vi "Plantilla.vi"() -> ()   [LabVIEW 2013]
uses:
  <vilib>/Platform/TimedLoop/XDataNode/timing_clust.ctl
  <vilib>/Platform/TimedLoop/XDataNode/nitl_modes.ctl
  <vilib>/Platform/TimedLoop/XDataNode/wakeup.ctl
  <vilib>/platform/TimedLoop/XDataNode/XDataNode.xnode
  <vilib>/Platform/TimedLoop/XDataNode/XDNodeRunTimeDep.lvlib
panel:
  out "Boolean 5":bool
  out "Boolean 4":bool
  in  "Offset Loop B 3":i64=5
  out "Boolean 3":bool
  out "Boolean 2":bool
  out "Boolean":bool
  in  "Offset Loop B 2":i64=5
  out "Timed Loop Iteration Start Times":i64[][](graph)
  in  "Offset Loop B":i64=5
  in  "Offset Loop A":i64
  in  "Period Loop A":i64=10
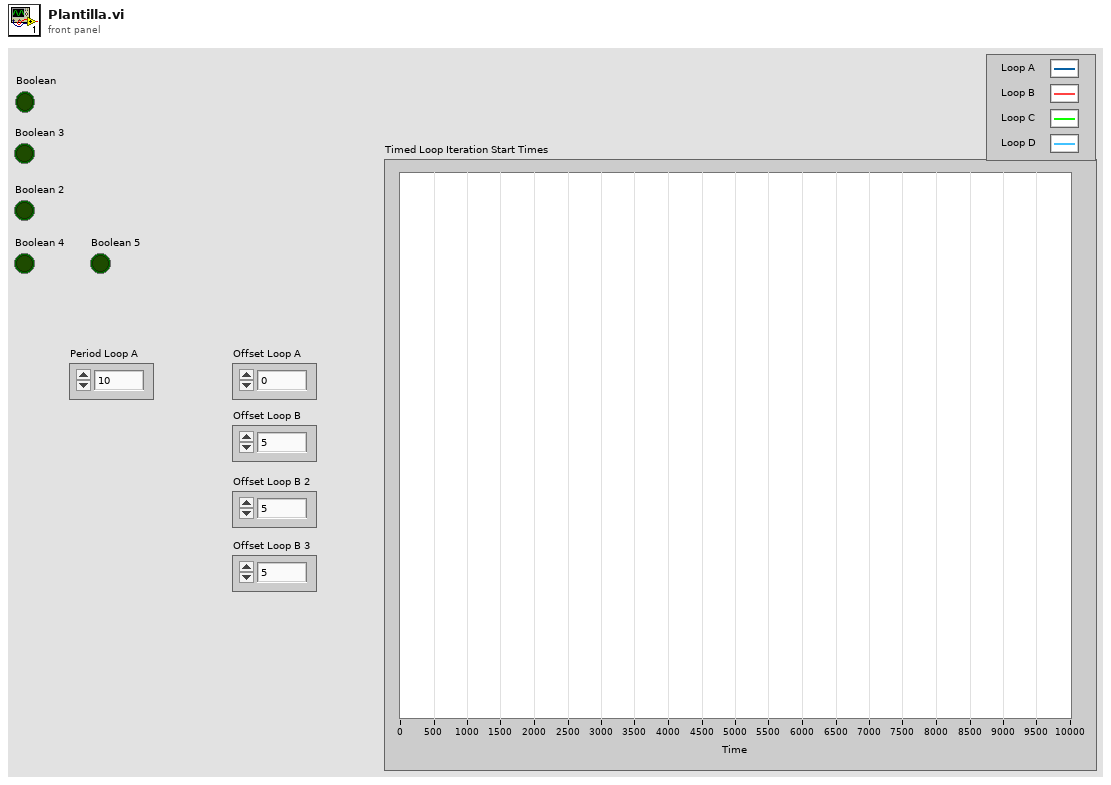
[diagram p1: front panel]
types:
  T1 = typedef "XDNodeRunTimeDep.lvlib/timing_clust.ctl" = cluster{"Expected End [f-1]":u64, "Actual End [f-1]":u64, "Finished Late? [f-1]":bool, "Expected End [i-1]":u64, "Actual End [i-1]":u64, "Finished Late? [i-1]":bool, "Expected Start [i]":u64, "Actual Start [i]":u64, "Expected Start [f]":u64, "Actual Start [f]":u64, "Source Name":string, "Structure Name":string, "Period":i64, "Deadline":i64, "Offset":i64, "Start":i64, "Priority":i32, "Timeout":i32, "Mode":T2, "Wakeup Reason":T3, "Error":errorcluster, "Source Type":string, "Secondary Source Type":string, "Global End Time":u64, "Global Start Time":u64, "Frame Duration":u64, "Iteration Duration":u64, "Assigned CPU":i32, "I/O Scan Engine Mode":u32}
  T2 = typedef "XDNodeRunTimeDep.lvlib/nitl_modes.ctl" = enum32{"No Change", "Process missed periods, maintain original phase", "Discard missed periods, maintain original phase", "Process missed periods, ignore original phase", "Discard missed periods, ignore original phase"}
  T3 = typedef "XDNodeRunTimeDep.lvlib/wakeup.ctl" = enum32{"Normal", "Aborted", "Asynchronous wakeup", "Timing source error", "Timed loop error", "Timeout"}
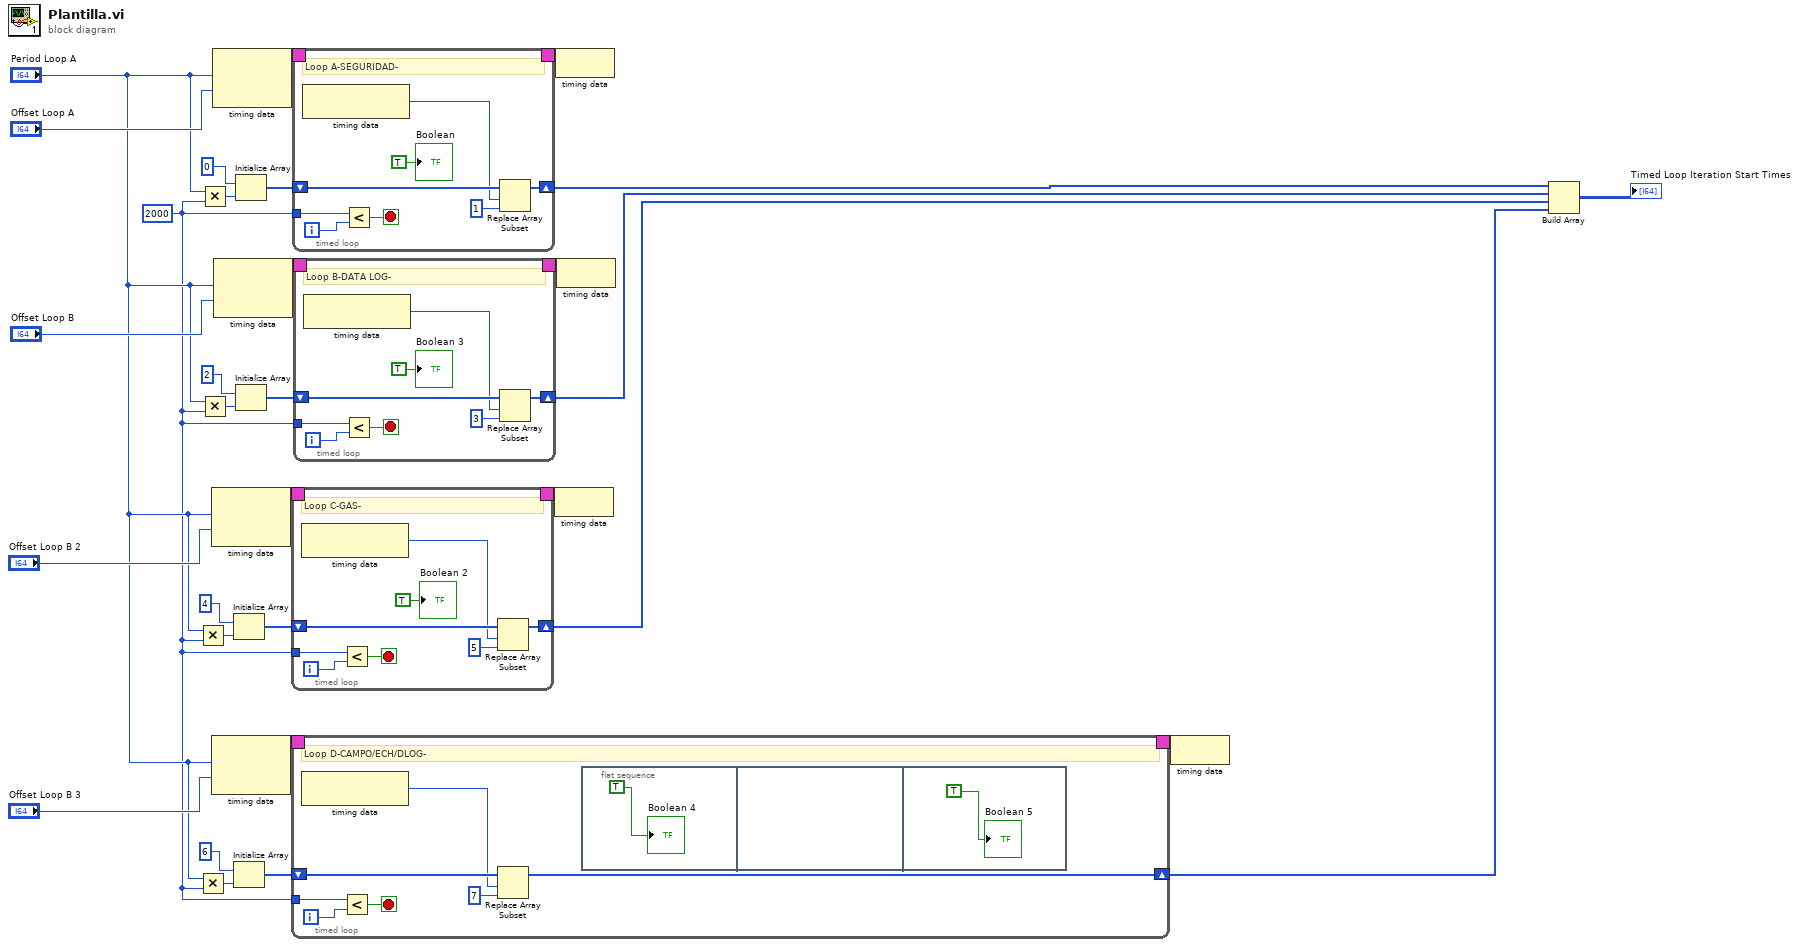
[diagram p0: block diagram]
diagram:
  w1 = i64 2000
  n1 = Multiply(x="Period Loop A", y=w1) -> (x*y=w13:i64)
  n2 = Multiply(x="Period Loop A", y=w1) -> (x*y=w6:i64)
  n3 = Multiply(x="Period Loop A", y=w1) -> (x*y=w25:i64)
  n4 = Multiply(x="Period Loop A", y=w1) -> (x*y=w22:i64)
  n5 = node-c288("Period Loop A", "Offset Loop B 2") -> (w16:T1)
  n6 = node-c288("Period Loop A", "Offset Loop B 3") -> (w9:T1)
  n7 = node-c288("Period Loop A", "Offset Loop A") -> (w29:T1)
  n8 = node-c288("Period Loop A", "Offset Loop B") -> (w31:T1)
  n9 = Initialize Array(i64 4, w13) -> (w12:i64[])
  n10 = Initialize Array(i64 6, w6) -> (w5:i64[])
  n11 = Initialize Array(i64 0, w25) -> (w24:i64[])
  n12 = Initialize Array(i64 2, w22) -> (w21:i64[])
  n13 = timed-loop {
    shift-left: w12 -> [w36]
    shift-right: [w34] -> w10
    tunnel: w1 -> [w37]
    timing-out: [_] -> w15
    timing: w16 -> [_]
    i -> [w39]
    stop <- w38 stop-if-true
    # "Loop C-GAS-"
    n14 = node-c288() -> (w33:i64)  [unwired: 1 in]
    n15 = Less?(x=w37, y=w39) -> (x < y?=w38:bool)
    n16 = Replace Array Subset(array=w36, new element=i64 5 ("new element/subarray"), index=w33) -> (w34:i64[])
    "Boolean 2" <- TRUE ("Boolean 2")
  }
  n17 = timed-loop {
    shift-left: w5 -> [w47]
    shift-right: [w45] -> w3
    timing-out: [_] -> w8
    timing: w9 -> [_]
    tunnel: w1 -> [w43]
    i -> [w49]
    stop <- w48 stop-if-true
    # "Loop D-CAMPO/ECH/DLOG-"
    n18 = node-c288() -> (w44:i64)  [unwired: 1 in]
    n19 = Less?(x=w43, y=w49) -> (x < y?=w48:bool)
    n20 = Replace Array Subset(array=w47, new element=i64 7 ("new element/subarray"), index=w44) -> (w45:i64[])
    n21 = flat-sequence {
      frame #0 {
        "Boolean 4" <- TRUE ("Boolean 2")
      }
      frame #1 {
      }
      frame #2 {
        "Boolean 5" <- TRUE ("Boolean 2")
      }
    }
  }
  n22 = timed-loop {
    shift-left: w24 -> [w59]
    shift-right: [w57] -> w18
    tunnel: w1 -> [w60]
    timing-out: [_] -> w28
    timing: w29 -> [_]
    i -> [w62]
    stop <- w61 stop-if-true
    # "Loop A-SEGURIDAD-"
    n23 = node-c288() -> (w56:i64)  [unwired: 1 in]
    n24 = Less?(x=w60, y=w62) -> (x < y?=w61:bool)
    n25 = Replace Array Subset(array=w59, new element=i64 1 ("new element/subarray"), index=w56) -> (w57:i64[])
    "Boolean" <- TRUE ("Boolean")
  }
  n26 = timed-loop {
    shift-left: w21 -> [w70]
    shift-right: [w68] -> w17
    tunnel: w1 -> [w71]
    timing-out: [_] -> w30
    timing: w31 -> [_]
    i -> [w73]
    stop <- w72 stop-if-true
    # "Loop B-DATA LOG-"
    n27 = node-c288() -> (w67:i64)  [unwired: 1 in]
    n28 = Less?(x=w71, y=w73) -> (x < y?=w72:bool)
    n29 = Replace Array Subset(array=w70, new element=i64 3 ("new element/subarray"), index=w67) -> (w68:i64[])
    "Boolean 3" <- TRUE ("Boolean 3")
  }
  n30 = node-c288(w15) -> ()
  n31 = node-c288(w28) -> ()
  n32 = node-c288(w30) -> ()
  n33 = node-c288(w8) -> ()
  n34 = Build Array(w18, w17, w10, w3) -> (→"Timed Loop Iteration Start Times":i64[][])
